vi "StartTest.vi"(8 "error in (no error)":errorcluster, 10 "TestCase":refnum<class "TestCase.lvclass">, 11 "TestListener in":refnum<class "TestListener.lvclass">) -> (0 "error out":errorcluster, 3 "TestListener out":refnum<class "TestListener.lvclass">)   [LabVIEW 2019, in "TestListener.lvclass"]
doc: "A test started."
uses:
  TestListener.lvclass
  TestCase/TestCase/TestCase.lvclass
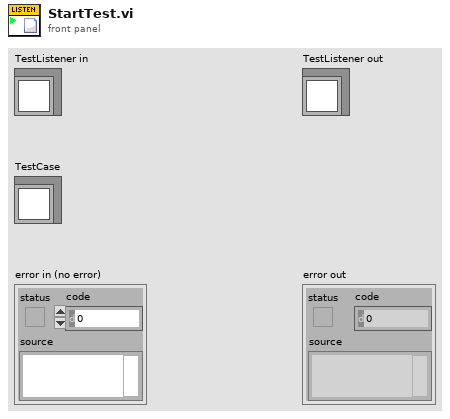
[diagram p1: front panel]
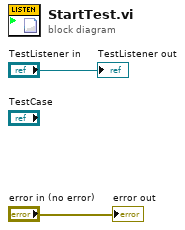
[diagram p0: block diagram]
diagram:
  "error out" <- "error in (no error)"
  "TestListener out" <- "TestListener in"
